vi "user process.vi"(8 "error in":errorcluster, 10 "ExampleStateMachine runtime in":refnum<class "ExampleStateMachine runtime.lvclass">, 11 "Parameters to process":T4) -> (0 "error out":errorcluster, 2 "ExampleStateMachine runtime out":refnum<class "ExampleStateMachine runtime.lvclass">, 3 "Results from processing":T3)   [LabVIEW 2017, in "ExampleStateMachine runtime.lvclass"]
uses:
  ExampleStateMachine runtime.lvclass
  parameter user data.ctl
  result user data.ctl
  Utilities/StateMachine.ctl
  Utilities/Results_Trajectory.ctl
  Utilities/Controlword_Commands.ctl
  CommandCluster.ctl
  Utilities/WordManipulationLibrary.lvlib
panel:
  out "Feedback":T1[](array[typedef])
  out "Status":T2
  out "Results":dbl[](array[numeric])
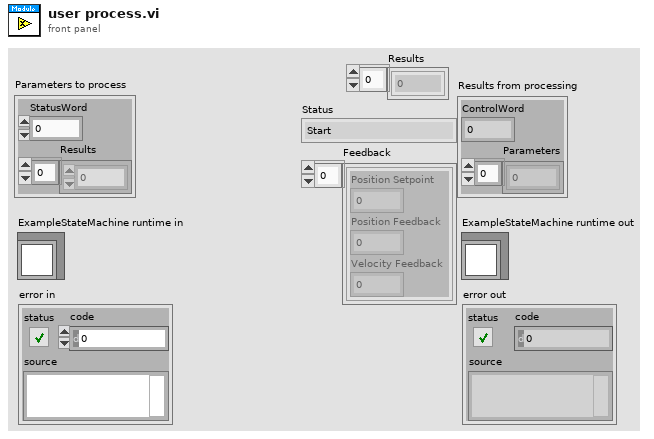
[diagram p1: front panel]
types:
  T1 = typedef "WordManipulationLibrary.lvlib/Results_Trajectory.ctl" = cluster{"Position Setpoint":dbl, "Position Feedback":dbl, "Velocity Feedback":dbl}
  T2 = typedef "WordManipulationLibrary.lvlib/StateMachine.ctl" = enum16{"Start", "Not Ready to Switch On", "Switch On Disabled", "Ready to Switch On", "Switched On", "Operation enable", "Quick Stop Active", "Fault Reaction Active", "Fault"}
  T3 = typedef "ExampleStateMachine runtime.lvclass/result user data.ctl" = cluster{"ControlWord":u16, "Parameters":dbl[]}
  T4 = typedef "ExampleStateMachine runtime.lvclass/parameter user data.ctl" = cluster{"StatusWord":u16, "Results":dbl[]}
  T5 = typedef "WordManipulationLibrary.lvlib/Controlword_Commands.ctl" = enum16{"Shutdown", "Switch On", "Disable Voltage", "Quick Stop", "Disable Op", "Enable Op", "Fault Reset", "Error"}
  T6 = enum16{"Shutdown", "Switch On", "Disable Voltage", "Quick Stop", "Disable Op", "Enable Op", "Fault Reset", "Error"}
  T7 = typedef "CommandCluster.ctl" = cluster{"Modes":enum16{"Reserved", "Profile Position Mode", "Velocity Mode", "Profile Velocity Mode", "Profile Torque Mode", "Reserved 2", "Reference Mode", "Interpolated Position Mode", "Skip"}, "Parameters_PositionProfile":dbl[]}
  T8 = enum16{"Reserved", "Profile Position Mode", "Velocity Mode", "Profile Velocity Mode", "Profile Torque Mode", "Reserved 2", "Reference Mode", "Interpolated Position Mode", "Skip"}
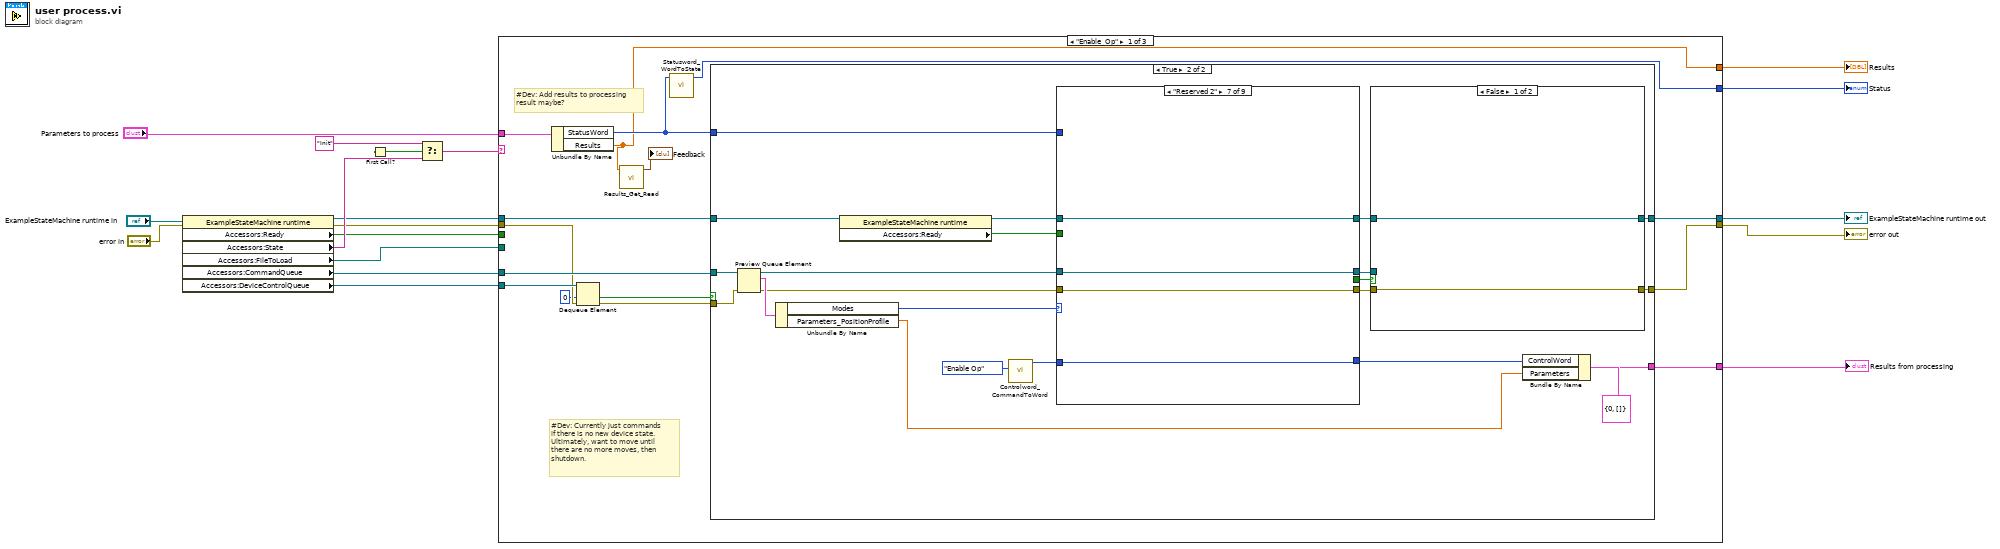
[diagram p0: block diagram]
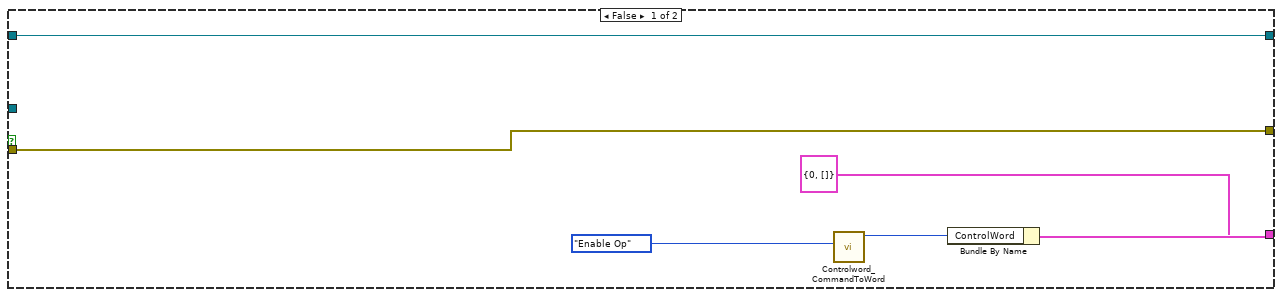
[diagram p2: hidden frame]
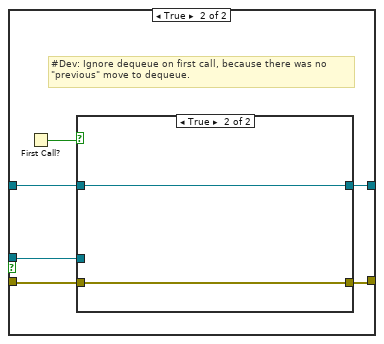
[diagram p3: hidden frame]
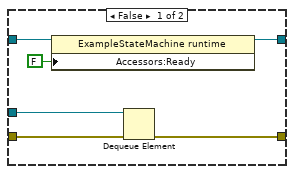
[diagram p4: hidden frame]
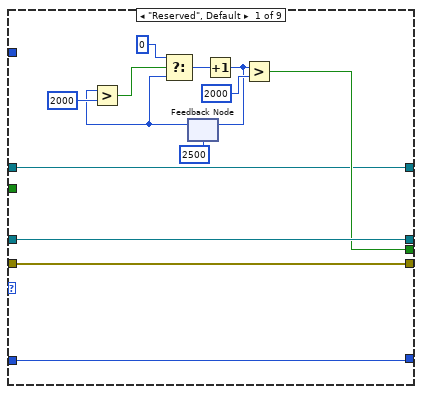
[diagram p5: hidden frame]
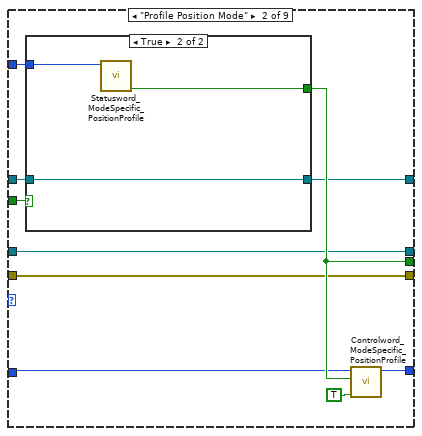
[diagram p6: hidden frame]
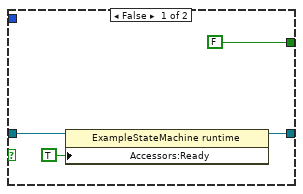
[diagram p7: hidden frame]
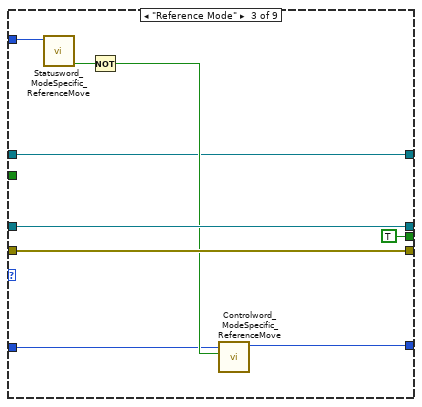
[diagram p8: hidden frame]
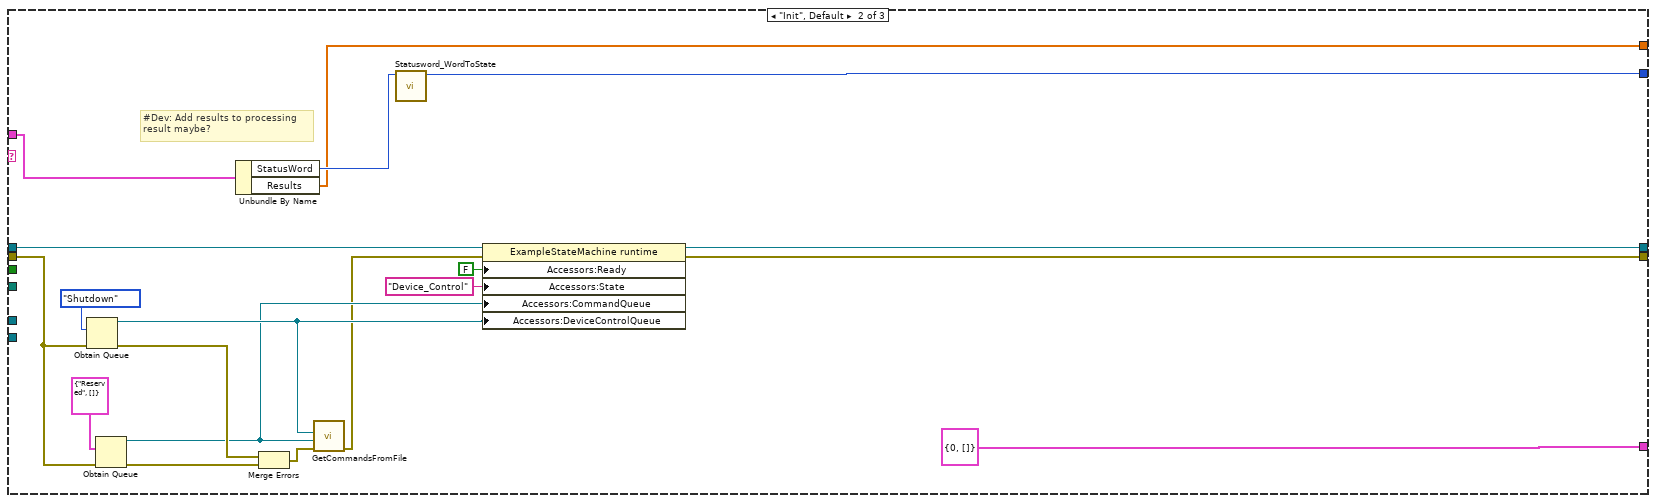
[diagram p14: hidden frame]
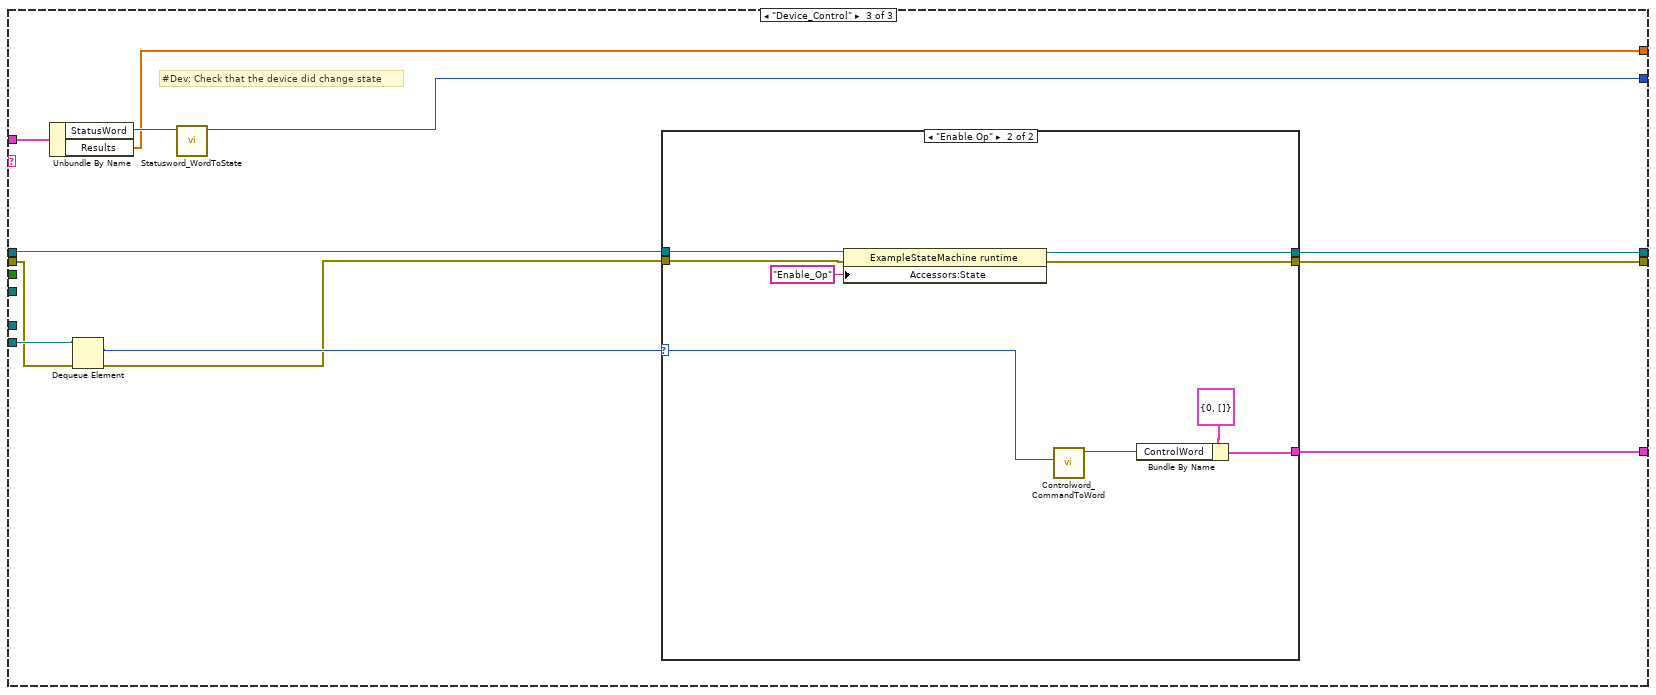
[diagram p15: hidden frame]
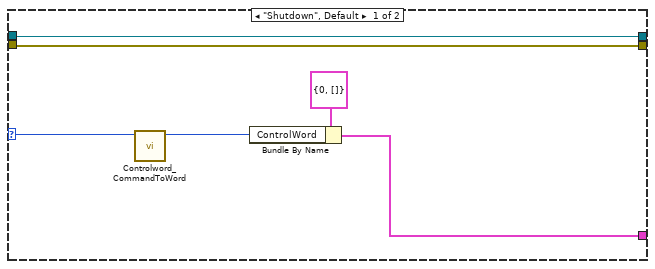
[diagram p16: hidden frame]
diagram:
  n1 = property class="ExampleStateMachine runtime"(reference="ExampleStateMachine runtime in", error in="error in") -> (reference out=w9:refnum<class "ExampleStateMachine runtime.lvclass">, error out=w7:errorcluster, "Accessors:Ready"=w5:bool, "Accessors:State"=w16:string, "Accessors:FileToLoad"=w10:path, "Accessors:CommandQueue"=w3:refnum<queue>, "Accessors:DeviceControlQueue"=w4:refnum<queue>)
  n2 = First Call?() -> (First Call?: T/F=w18:bool)
  n3 = Select(t="Init" ("f"), s=w18, f=w16) -> (s? t:f=w13:string)
  n4 = case shown="\"Enable_Op\"" w13 {
    tunnel: "Parameters to process" -> [w27 w143 w169]
    tunnel: [w28 T3 {"ControlWord"=0, "Parameters"=[]} ("Results from processing") w171] -> w11
    tunnel: w10 -> [_ _ _]
    tunnel: w9 -> [w32 w158 w170]
    tunnel: [w25 w157 w165] -> w8
    tunnel: w7 -> [w30 w154 w164]
    tunnel: [w26 w156 w162] -> w6
    tunnel: w5 -> [_ _ _]
    tunnel: w4 -> [w33 _ w167]
    tunnel: w3 -> [w31 _ _]
    tunnel: [w23 w142 w161] -> w2
    tunnel: [w22 w141 w160] -> w1
    frame "Enable_Op" {
      # "#Dev: Add results to processing\nresult maybe?"
      # "#Dev: Currently just commands\nif there is no new device state.\nUltimately, want to move until\nthere are no more moves, then\nshutdown."
      n5 = Unbundle By Name(w27) -> ("StatusWord"=w24:u16, "Results"=w22:dbl[])
      n6 = Dequeue Element(queue=w33, timeout in ms (-1)=0, error in (no error)=w30) -> (timed out?=w19:bool, error out=w29:errorcluster)  [unwired: 2 out]
      n7 = call "Results_Get_Read.vi"("appended array"=w22) -> ("Feedback"=→"Feedback":T1[])  [unwired: 8 in, 2 out]
      n8 = call "Statusword_WordToState.vi"("Data_In"=w24) -> ("Status"=w23:T2)  [unwired: 10 in]
      n9 = case shown="True" w19 {
        tunnel: w32 -> [w39 w46]
        tunnel: w31 -> [_ w57]
        tunnel: w29 -> [w38 w58]
        tunnel: [w36 w59] -> w28
        tunnel: w24 -> [_ w55]
        tunnel: [w38 w47] -> w26
        tunnel: [w39 w40] -> w25
        frame False {
          n10 = call "Controlword_CommandToWord.vi"("Device Control Command"=Controlword_Commands."Enable Op") -> ("ControlWord Out"=w34:u16)  [unwired: 10 in]
          n11 = Bundle By Name(cluster=T3 {"ControlWord"=0, "Parameters"=[]} ("Results from processing"), "ControlWord"=w34) -> (w36:T3)
        }
        frame True {
          n12 = Preview Queue Element(queue=w57, error in (no error)=w58) -> (queue out=w54:refnum<queue>, element=w56:T7, error out=w53:errorcluster)  [unwired: 1 in, 1 out]
          n13 = Unbundle By Name(w56) -> ("Modes"=w50:T8, "Parameters_PositionProfile"=w42:dbl[])
          n14 = property class="ExampleStateMachine runtime"(reference=w46) -> (reference out=w44:refnum<class "ExampleStateMachine runtime.lvclass">, "Accessors:Ready"=w45:bool)  [unwired: 1 in, 1 out]
          n15 = call "Controlword_CommandToWord.vi"("Device Control Command"=Controlword_Commands."Enable Op") -> ("ControlWord Out"=w48:u16)  [unwired: 10 in]
          n16 = case shown="\"Reserved 2\"" w50 {
            tunnel: [w88 w99 w111 w118 w122 w126 w130 w134 w138] -> w61
            tunnel: w55 -> [_ w98 w113 _ _ _ _ _ _]
            tunnel: w54 -> [w90 w94 w116 w120 w124 w128 w132 w136 w140]
            tunnel: w53 -> [w89 w93 w115 w119 w123 w127 w131 w135 w139]
            tunnel: [w90 w94 w116 w120 w124 w128 w132 w136 w140] -> w52
            tunnel: [w89 w93 w115 w119 w123 w127 w131 w135 w139] -> w51
            tunnel: w48 -> [w88 w92 w110 w118 w122 w126 w130 w134 w138]
            tunnel: w45 -> [_ w97 _ _ _ _ _ _ _]
            tunnel: w44 -> [w79 w96 w108 w117 w121 w125 w129 w133 w137]
            tunnel: [w84 w95 TRUE ("Set Point Reached?") _ _ _ _ _ _] -> w43
            tunnel: [w79 w91 w108 w117 w121 w125 w129 w133 w137] -> w41
            frame "Reserved", Default {
              n17 = feedback #1(2500) -> (w80:i32)
              n18 = Greater?(x=w80, y=2000) -> (0:w81:bool)
              n19 = Select(t=0, s=w81, f=w80) -> (s? t:f=w85:i32)
              n20 = Increment(x=w85) -> (x+1=w83:i32)
              n21 = feedback-in #1(w83) -> ()
              n22 = Greater?(x=w83, y=2000) -> (0:w84:bool)
            }
            frame "Profile Position Mode" {
              n23 = case shown="True" w97 {
                tunnel: w98 -> [_ w107]
                tunnel: [FALSE ("Set Point Reached?") w106] -> w95
                tunnel: w96 -> [w103 w105]
                tunnel: [w101 w105] -> w91
                frame False {
                  n24 = property class="ExampleStateMachine runtime"(reference=w103, "Accessors:Ready"=TRUE ("Ready")) -> (reference out=w101:refnum<class "ExampleStateMachine runtime.lvclass">)  [unwired: 1 in, 1 out]
                }
                frame True {
                  n25 = call "Statusword_ModeSpecific_PositionProfile.vi"("StatusWord In"=w107) -> ("Set Point Reached?"=w106:bool)  [unwired: 7 in, 3 out]
                }
              }
              n26 = call "Controlword_ModeSpecific_PositionProfile.vi"("Relative?"=TRUE ("Absolute?"), "New Setpoint?"=w95, "ControlWord In"=w92) -> ("ControlWord Out"=w99:u16)  [unwired: 8 in]
            }
            frame "Reference Mode" {
              n27 = call "Statusword_ModeSpecific_ReferenceMove.vi"("StatusWord In"=w113) -> ("Set Point Reached?"=w114:bool)  [unwired: 9 in, 1 out]
              n28 = Not(x=w114) -> (.not. x?=w112:bool)
              n29 = call "Controlword_ModeSpecific_ReferenceMove.vi"("Operation Start"=w112, "ControlWord In"=w110) -> ("ControlWord Out"=w111:u16)  [unwired: 9 in]
            }
            frame "Velocity Mode" {
            }
            frame "Profile Velocity Mode" {
            }
            frame "Profile Torque Mode" {
            }
            frame "Reserved 2" {
            }
            frame "Interpolated Position Mode" {
            }
            frame "Skip" {
            }
          }
          n30 = case shown="False" w43 {
            tunnel: w52 -> [_ w67]
            tunnel: w51 -> [w63 w69]
            tunnel: [w63 w68] -> w47
            tunnel: w41 -> [w62 w66]
            tunnel: [w62 w65] -> w40
            frame False {
            }
            frame True {
              # "#Dev: Ignore dequeue on first call, because there was no \n\"previous\" move to dequeue."
              n31 = First Call?() -> (First Call?: T/F=w64:bool)
              n32 = case shown="True" w64 {
                tunnel: w69 -> [w75 w76]
                tunnel: [w74 w76] -> w68
                tunnel: w67 -> [w73 _]
                tunnel: w66 -> [w72 w77]
                tunnel: [w71 w77] -> w65
                frame False {
                  n33 = property class="ExampleStateMachine runtime"(reference=w72, "Accessors:Ready"=FALSE ("Ready")) -> (reference out=w71:refnum<class "ExampleStateMachine runtime.lvclass">)  [unwired: 1 in, 1 out]
                  n34 = Dequeue Element(queue=w73, error in (no error)=w75) -> (error out=w74:errorcluster)  [unwired: 1 in, 3 out]
                }
                frame True {
                }
              }
            }
          }
          n35 = Bundle By Name(cluster=T3 {"ControlWord"=0, "Parameters"=[]} ("Results from processing"), "ControlWord"=w61, "Parameters"=w42) -> (w59:T3)
        }
      }
    }
    frame "Init", Default {
      # "#Dev: Add results to processing\nresult maybe?"
      n36 = Obtain Queue(element data type=T6."Shutdown" ("Device Control Command"), error in (no error)=w154) -> (queue out=w147:refnum<queue>, error out=w149:errorcluster)  [unwired: 3 in, 1 out]
      n37 = Obtain Queue(element data type=T7 {"Modes"=enum."Reserved", "Parameters_PositionProfile"=[]}, error in (no error)=w154) -> (queue out=w146:refnum<queue>, error out=w150:errorcluster)  [unwired: 3 in, 1 out]
      n38 = Unbundle By Name(w143) -> ("StatusWord"=w144:u16, "Results"=w141:dbl[])
      n39 = Merge Errors(w149, w150) -> (w148:errorcluster)
      n40 = call "GetCommandsFromFile.vi"("error in"=w148, "CommandQueue"=w146, "DeviceControlQueue"=w147) -> ("error out"=w145:errorcluster)  [unwired: 8 in]
      n41 = call "Statusword_WordToState.vi"("Data_In"=w144) -> ("Status"=w142:T2)  [unwired: 10 in]
      n42 = property class="ExampleStateMachine runtime"(reference=w158, error in=w145, "Accessors:Ready"=FALSE ("Running"), "Accessors:State"="Device_Control" ("State"), "Accessors:CommandQueue"=w146, "Accessors:DeviceControlQueue"=w147) -> (reference out=w157:refnum<class "ExampleStateMachine runtime.lvclass">, error out=w156:errorcluster)
    }
    frame "Device_Control" {
      # "#Dev: Check that the device did change state"
      n43 = Unbundle By Name(w169) -> ("StatusWord"=w168:u16, "Results"=w160:dbl[])
      n44 = Dequeue Element(queue=w167, error in (no error)=w164) -> (element=w166:T6, error out=w163:errorcluster)  [unwired: 1 in, 2 out]
      n45 = call "Statusword_WordToState.vi"("Data_In"=w168) -> ("Status"=w161:T2)  [unwired: 10 in]
      n46 = case shown="\"Enable Op\"" w166 {
        selector: w166 -> [w174 w178]
        tunnel: [w175 w179] -> w171
        tunnel: w170 -> [w173 w186]
        tunnel: [w173 w185] -> w165
        tunnel: w163 -> [w172 w183]
        tunnel: [w172 w182] -> w162
        frame "Shutdown", Default {
          n47 = call "Controlword_CommandToWord.vi"("ControlWord In"=w174) -> ("ControlWord Out"=w176:u16)  [unwired: 10 in]
          n48 = Bundle By Name(cluster=T3 {"ControlWord"=0, "Parameters"=[]} ("Results from processing"), "ControlWord"=w176) -> (w175:T3)
        }
        frame "Enable Op" {
          n49 = property class="ExampleStateMachine runtime"(reference=w186, error in=w183, "Accessors:State"="Enable_Op" ("State")) -> (reference out=w185:refnum<class "ExampleStateMachine runtime.lvclass">, error out=w182:errorcluster)
          n50 = call "Controlword_CommandToWord.vi"("Device Control Command"=w178) -> ("ControlWord Out"=w181:u16)  [unwired: 10 in]
          n51 = Bundle By Name(cluster=T3 {"ControlWord"=0, "Parameters"=[]} ("Results from processing"), "ControlWord"=w181) -> (w179:T3)
        }
      }
    }
  }
  "error out" <- w6
  "Results from processing" <- w11
  "ExampleStateMachine runtime out" <- w8
  "Status" <- w2
  "Results" <- w1
